vi "基于LabVIEW的风电机组故障诊断.vi"() -> ()   [LabVIEW 2018]
uses:
  <vilib>/Analysis/baseanly.llb/Mean (DBL).vi
  <vilib>/Analysis/2dsp.llb/Real FFT.vi
  <vilib>/Analysis/5stat.llb/RMS (DBL).vi
  <vilib>/Analysis/2dsp.llb/Inverse Real FFT.vi
  <vilib>/Utility/file.llb/Read From Spreadsheet File (DBL).vi
  <vilib>/Analysis/3filter.llb/Equi-Ripple BandStop (DBL).vi
  <vilib>/Analysis/NI_AALPro.lvlib
  <vilib>/Analysis/NI_AALBase.lvlib
  <vilib>/gmath/NI_Gmath.lvlib
panel:
  in  "布尔":bool
  out "位置":string
  in  "采样频率1":dbl=2000.0 format="%0.2f"
  in  "相关系数路径":path=path "C:/Documents and Settings/Administrator/桌面/zhengchang1480.txt"
  in  "测点号 2":i32=1
  out "相关系数":dbl=1.742594479126076
  out "峭度":dbl=2.3271834018013804
  out "有效值":dbl
  out "峰峰值":dbl
  in  "?":T1(tab)
  out "时域波形图":waveform(dbl)(graph)={"t0"=timestamp(0 s since 1904-01-01), "dt"=0.0001953125, "Y"=array[4096 elements]}
  out "解调后波形图":waveform(dbl)(graph)={"t0"=timestamp(0 s since 1904-01-01), "dt"=0.0001953125, "Y"=array[4096 elements]}
  out "倒谱":waveform(dbl)(graph)={"t0"=timestamp(0 s since 1904-01-01), "dt"=0.000390625, "Y"=array[2048 elements]}
  out "频谱图":cluster{"x":i32, dbl, dbl[]}(graph)
  out "包络谱":cluster{"x":i32, dbl, dbl[]}(graph)
  in  "采样频率":dbl=5120.0
  in  "测点号":i32=1
  in  "文件读取路径":path=path "C:/Documents and Settings/Administrator/桌面/zhengchang1480.txt"
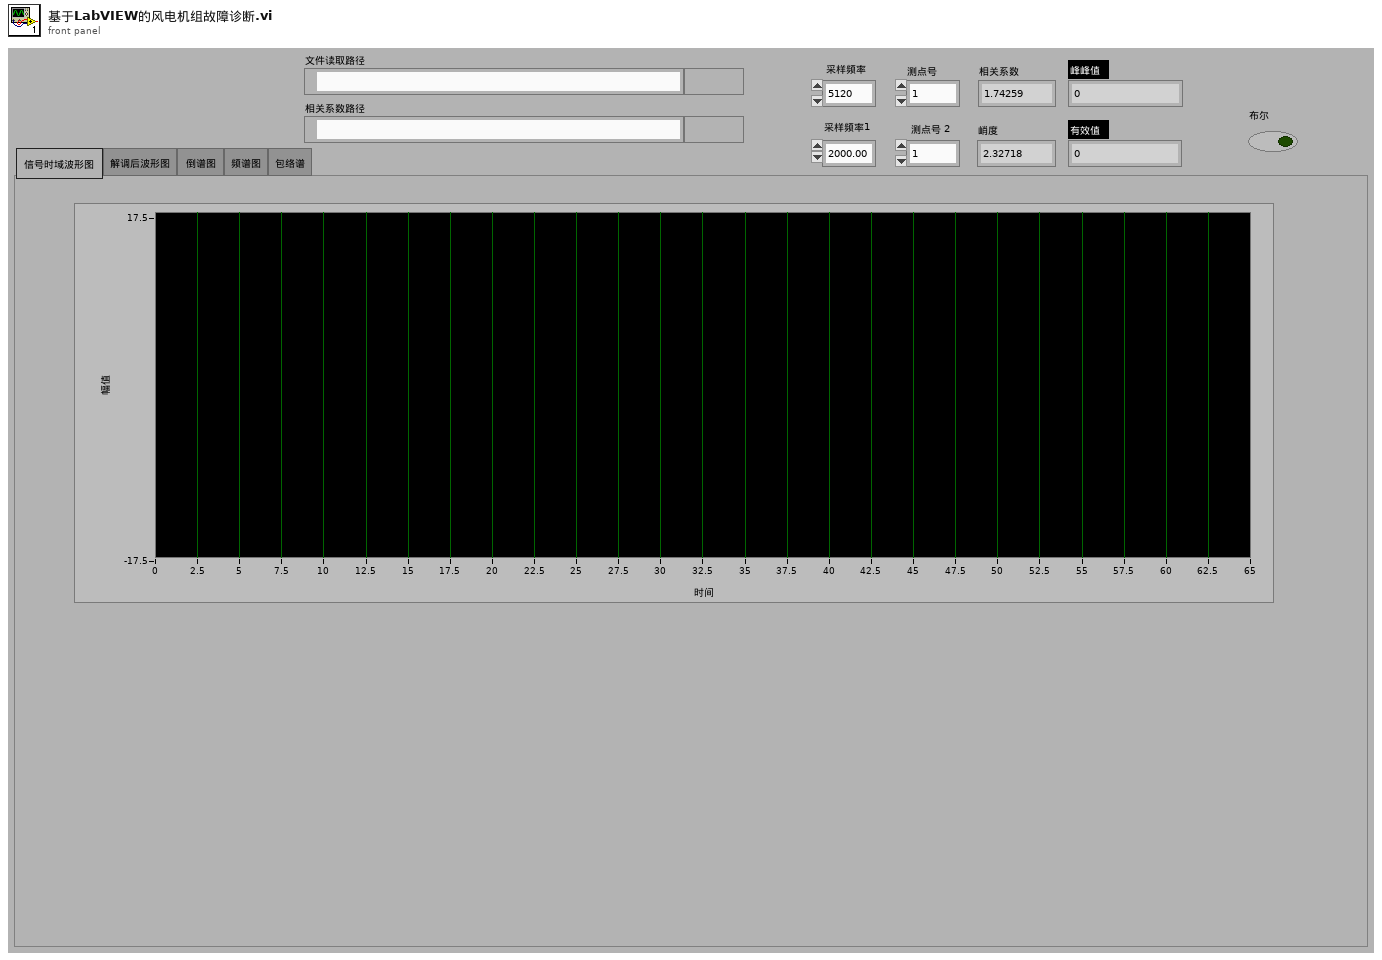
[diagram p1: front panel]
types:
  T1 = enum32{"信号时域波形图 ", "解调后波形图", "倒谱图 ", "频谱图", "包络谱"}
  T2 = typedef "LVPoint32TypeDef.ctl" = cluster{"Horizontal":i32, "Vertical":i32}
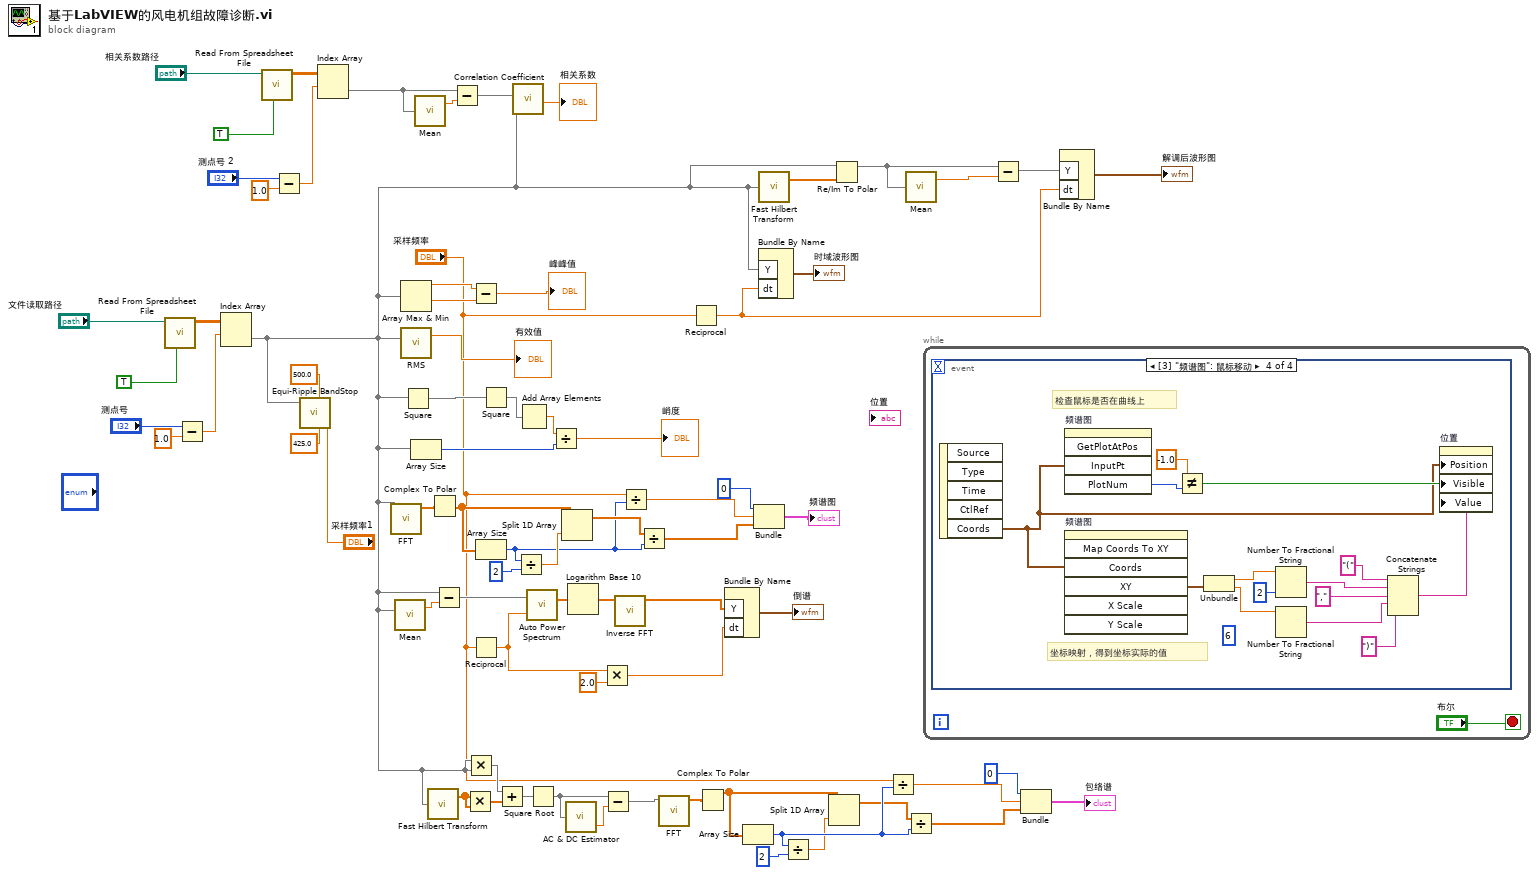
[diagram p0: block diagram]
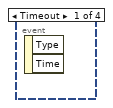
[diagram p2: hidden frame]
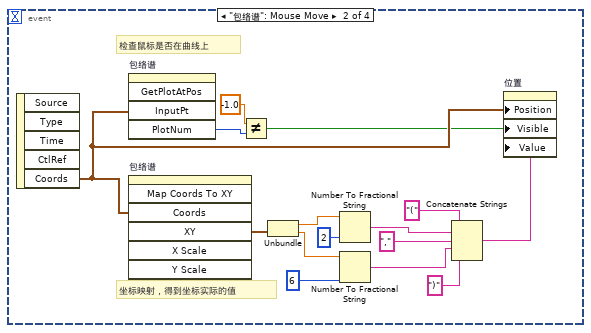
[diagram p3: hidden frame]
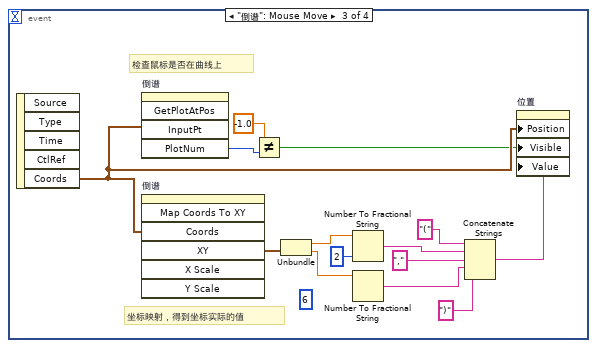
[diagram p4: hidden frame]
diagram:
  n1 = call-poly <vilib>:"Read From Spreadsheet File.vi"("transpose (no:F)"=TRUE, "file path (dialog if empty)"="文件读取路径") -> ("all rows"=w71:dbl[][])  [unwired: 5 in, 4 out]
  n2 = Subtract(x="测点号", y=1.0) -> (x-y=w68:dbl)
  n3 = Index Array(array=w71, index (row)=w68) -> (element=w13:dbl[])  [unwired: 1 in]
  n4 = call-poly <vilib>:"Read From Spreadsheet File.vi"("transpose (no:F)"=TRUE, "file path (dialog if empty)"="相关系数路径") -> ("all rows"=w54:dbl[][])  [unwired: 5 in, 4 out]
  n5 = Subtract(x="测点号 2", y=1.0) -> (x-y=w58:dbl)
  n6 = call-poly <vilib>:"Equi-Ripple BandStop.vi"("X"=w13, "higher pass freq"=500.0, "higher stop freq"=425.0, "sampling freq: fs"="采样频率1") -> ()  [unwired: 4 in, 2 out]
  n7 = Index Array(array=w54, index (row)=w58) -> (element=w60:dbl[])  [unwired: 1 in]
  n8 = call-poly <vilib>:"FFT.vi"("X"=w13) -> ("FFT {X}"=w28:cdb[])  [unwired: 9 in, 1 out]
  n9 = call-poly <vilib>:"Mean.vi"("X"=w13) -> ("mean"=w26:dbl)  [unwired: 1 out]
  n10 = Array Max & Min(array=w13) -> (max value=w50:dbl, min value=w49:dbl)  [unwired: 2 out]
  n11 = call-poly <vilib>:"RMS.vi"("X"=w13) -> ("rms value"=→"有效值":dbl)  [unwired: 1 out]
  n12 = Square(x=w13) -> (x^2=w64:dbl[])
  n13 = Array Size(array=w13) -> (size(s)=w29:i32)
  n14 = call-poly <vilib>:"Mean.vi"("X"=w60) -> ("mean"=w56:dbl)  [unwired: 1 out]
  n15 = call <vilib>:"Fast Hilbert Transform.vi"("X"=w13) -> ("Hilbert{X}"=w18:dbl[])  [unwired: 1 out]
  n16 = Complex To Polar(r * e^(i*theta)=w28) -> (r=w46:dbl[])  [unwired: 1 out]
  n17 = Subtract(x=w13, y=w26) -> (x-y=w24:dbl[])
  n18 = Subtract(x=w60, y=w56) -> (x-y=w52:dbl[])
  n19 = Multiply(x=w18, y=w18) -> (x*y=w17:dbl[])
  n20 = Multiply(x=w13, y=w13) -> (x*y=w19:dbl[])
  n21 = Subtract(x=w50, y=w49) -> (x-y=→"峰峰值":dbl)
  n22 = Reciprocal(x="采样频率") -> (1/x=w22:dbl)
  n23 = Array Size(array=w46) -> (size(s)=w42:i32)
  n24 = Square(x=w64) -> (x^2=w63:dbl[])
  n25 = Add(x=w19, y=w17) -> (x+y=w16:dbl[])
  n26 = call <vilib>:"Correlation Coefficient.vi"("Y"=w52, "X"=w13) -> ("correlation coefficient r"=→"相关系数":dbl)  [unwired: 8 in, 1 out]
  n27 = Divide(x=w42, y=2 ("x")) -> (x/y=w44:dbl)
  n28 = Add Array Elements(numeric array=w63) -> (sum=w30:dbl)
  n29 = call <vilib>:"Auto Power Spectrum.vi"("dt"=w22, "Signal (V)"=w24) -> ("Power Spectrum (V^2 rms)"=w27:dbl[])  [unwired: 1 out]
  n30 = Square Root(x=w16) -> (sqrt(x)=w15:dbl[])
  n31 = Divide(x=w30, y=w29) -> (x/y=→"峭度":dbl)
  n32 = Split 1D Array(array=w46, index=w44) -> (first subarray=w47:dbl[])  [unwired: 1 out]
  n33 = call <vilib>:"AC & DC Estimator.vi"("Signal (V)"=w15) -> ("DC estimate (V)"=w14:dbl)  [unwired: 1 out]
  n34 = Logarithm Base 10(1:w27) -> (0:w25:dbl[])
  n35 = Multiply(x=w22, y=2.0) -> (x*y=w21:dbl)
  n36 = Subtract(x=w15, y=w14) -> (x-y=w3:dbl[])
  n37 = call-poly <vilib>:"Inverse FFT.vi"("FFT {X}"=w25) -> ("X"=w23:dbl[])  [unwired: 9 in, 1 out]
  n38 = Divide(x="采样频率", y=w42) -> (x/y=w41:dbl)
  n39 = Divide(x=w47, y=w42) -> (x/y=w43:dbl[])
  n40 = call-poly <vilib>:"FFT.vi"("X"=w3) -> ("FFT {X}"=w12:cdb[])  [unwired: 9 in, 1 out]
  n41 = Reciprocal(x="采样频率") -> (1/x=w35:dbl)
  n42 = Complex To Polar(r * e^(i*theta)=w12) -> (r=w5:dbl[])  [unwired: 1 out]
  n43 = Bundle By Name("Y"=w23, "dt"=w21) -> (→"倒谱":waveform(dbl))  [unwired: 1 in]
  n44 = Array Size(array=w5) -> (size(s)=w9:i32)
  n45 = Bundle("x"=0, w41, w43) -> (→"频谱图":cluster{"x":i32, dbl, dbl[]})  [unwired: 1 in]
  n46 = call <vilib>:"Fast Hilbert Transform.vi"("X"=w13) -> ("Hilbert{X}"=w73:dbl[])  [unwired: 1 out]
  n47 = Bundle By Name("Y"=w13, "dt"=w35) -> (→"时域波形图":waveform(dbl))  [unwired: 1 in]
  n48 = Divide(x=w9, y=2 ("x")) -> (x/y=w7:dbl)
  n49 = Split 1D Array(array=w5, index=w7) -> (first subarray=w4:dbl[])  [unwired: 1 out]
  n50 = Re/Im To Polar(2:w73, 3:w13) -> (1:w36:dbl[])  [unwired: 1 out]
  n51 = Divide(x="采样频率", y=w9) -> (x/y=w10:dbl)
  n52 = call-poly <vilib>:"Mean.vi"("X"=w36) -> ("mean"=w65:dbl)  [unwired: 1 out]
  n53 = Divide(x=w4, y=w9) -> (x/y=w8:dbl[])
  n54 = while {
    stop <- "布尔" stop-if-true
    n55 = event shown="[3] \"频谱图\": 鼠标移动" {
      selector: _ -> [_ _ _ _]
      dyn-events: _ -> [_ _ _ _]
      timeout: _ -> [_ _ _ _]
      event Timeout {
        n56 = event-data() -> ()  [unwired: 1 in, 2 out]
      }
      event "包络谱": Mouse Move {
        # "坐标映射，得到坐标实际的值"
        # "检查鼠标是否在曲线上"
        n57 = event-data() -> ("Coords"=w77:T2)  [unwired: 1 in, 4 out]
        n58 = invoke on="包络谱" class="WFGraph (严格)" method="GetPlotAtPos"("InputPt"=w77) -> ("PlotNum"=w85:i32)  [unwired: 4 in, 4 out]
        n59 = invoke on="包络谱" class="WFGraph (严格)" method="Map Coords To XY"("Coords"=w77) -> ("XY"=w86:cluster{"X":dbl, "Y":dbl})  [unwired: 6 in, 6 out]
        n60 = Not Equal?(x=-1.0 ("y"), y=w85) -> (x != y?=w76:bool)
        n61 = Unbundle(w86) -> ("X"=w87:dbl, "Y"=w88:dbl)
        n62 = Number To Fractional String(number=w87, precision (6)=i16 2) -> (F-format string=w89:string)  [unwired: 2 in]
        n63 = Number To Fractional String(number=w88, precision (6)=i16 6) -> (F-format string=w82:string)  [unwired: 2 in]
        n64 = Concatenate Strings("(", w89, ",", w82, ")") -> (w75:string)
        n65 = property on="位置" class="Str"("Position"=w77, "Visible"=w76, "Value"=w75) -> ()  [unwired: 2 in, 2 out]
      }
      event "倒谱": Mouse Move {
        (unwired) i16 6 ("precision (6)")
        # "坐标映射，得到坐标实际的值"
        # "检查鼠标是否在曲线上"
        n66 = event-data() -> ("Coords"=w92:T2)  [unwired: 1 in, 4 out]
        n67 = invoke on="倒谱" class="WFGraph (严格)" method="GetPlotAtPos"("InputPt"=w92) -> ("PlotNum"=w102:i32)  [unwired: 4 in, 4 out]
        n68 = invoke on="倒谱" class="WFGraph (严格)" method="Map Coords To XY"("Coords"=w92) -> ("XY"=w101:cluster{"X":dbl, "Y":dbl})  [unwired: 6 in, 6 out]
        n69 = Not Equal?(x=-1.0 ("y"), y=w102) -> (x != y?=w91:bool)
        n70 = Unbundle(w101) -> ("X"=w100:dbl, "Y"=w99:dbl)
        n71 = Number To Fractional String(number=w100, precision (6)=i16 2) -> (F-format string=w98:string)  [unwired: 2 in]
        n72 = Number To Fractional String(number=w99) -> (F-format string=w103:string)  [unwired: 3 in]
        n73 = Concatenate Strings("(", w98, ",", w103, ")") -> (w90:string)
        n74 = property on="位置" class="Str"("Position"=w92, "Visible"=w91, "Value"=w90) -> ()  [unwired: 2 in, 2 out]
      }
      event "频谱图": Mouse Move {
        (unwired) i16 6 ("precision (6)")
        # "坐标映射，得到坐标实际的值"
        # "检查鼠标是否在曲线上"
        n75 = event-data() -> ("Coords"=w104:T2)  [unwired: 1 in, 4 out]
        n76 = invoke on="频谱图" class="WFGraph (严格)" method="GetPlotAtPos"("InputPt"=w104) -> ("PlotNum"=w111:i32)  [unwired: 4 in, 4 out]
        n77 = invoke on="频谱图" class="WFGraph (严格)" method="Map Coords To XY"("Coords"=w104) -> ("XY"=w112:cluster{"X":dbl, "Y":dbl})  [unwired: 6 in, 6 out]
        n78 = Not Equal?(x=-1.0 ("y"), y=w111) -> (x != y?=w116:bool)
        n79 = Unbundle(w112) -> ("X"=w113:dbl, "Y"=w114:dbl)
        n80 = Number To Fractional String(number=w113, precision (6)=i16 2) -> (F-format string=w115:string)  [unwired: 2 in]
        n81 = Number To Fractional String(number=w114) -> (F-format string=w110:string)  [unwired: 3 in]
        n82 = Concatenate Strings("(", w115, ",", w110, ")") -> (w117:string)
        n83 = property on="位置" class="Str"("Position"=w104, "Visible"=w116, "Value"=w117) -> ()  [unwired: 2 in, 2 out]
      }
    }
  }
  n84 = Subtract(x=w36, y=w65) -> (x-y=w37:dbl[])
  n85 = Bundle("x"=0, w10, w8) -> (→"包络谱":cluster{"x":i32, dbl, dbl[]})  [unwired: 1 in]
  n86 = Bundle By Name("Y"=w37, "dt"=w35) -> (→"解调后波形图":waveform(dbl))  [unwired: 1 in]
